vi "Get systemMetrics.vi"(8 "error in":errorcluster) -> (0 "error out":errorcluster, 1 "height":u32, 2 "width":u32)   [LabVIEW 2012]
uses:
  C:/Windows/System32/user32.dll
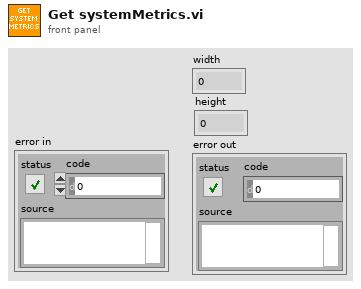
[diagram p1: front panel]
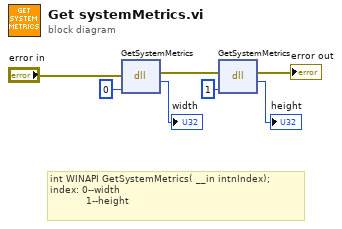
[diagram p0: block diagram]
diagram:
  # "int WINAPI GetSystemMetrics( __in intnIndex);\nindex: 0--width\n            1--height"
  n1 = dll-call lib="C:/Windows/System32/user32.dll" fn="GetSystemMetrics"(error in="error in", "arg1"=u32 0) -> (error out=w1:errorcluster, "return type"=→"width":u32)  [unwired: 3 in, 1 out]
  n2 = dll-call lib="C:/Windows/System32/user32.dll" fn="GetSystemMetrics"(error in=w1, "arg1"=u32 1) -> (error out=→"error out":errorcluster, "return type"=→"height":u32)  [unwired: 3 in, 1 out]
